vi "Event Loop Async.vi"(10 "Handshake":refnum<notifier>, 11 "ControlArray in":refnum<class "ControlArray.lvclass">) -> ()   [LabVIEW 2020, in "Control Array.lvlib" / "ControlArray.lvclass"]
uses:
  ControlArray.lvclass
  ControlArray.lvclass/ControlArray.ctl
  Element Changed Event Data.ctl
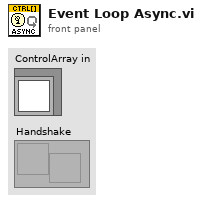
[diagram p1: front panel]
types:
  T1 = typedef "Control Array.lvlib/ControlArray.lvclass/Events.ctl" = cluster{"Stop":refnum<user-event>, "Remove Element":refnum<user-event>, "Add Element":refnum<user-event>}
  T2 = typedef "Control Array.lvlib/ControlArray.lvclass/Element Changed Event Data.ctl" = cluster{"Value":variant, "Index":i32, "Ctl Ref":refnum<vi>}
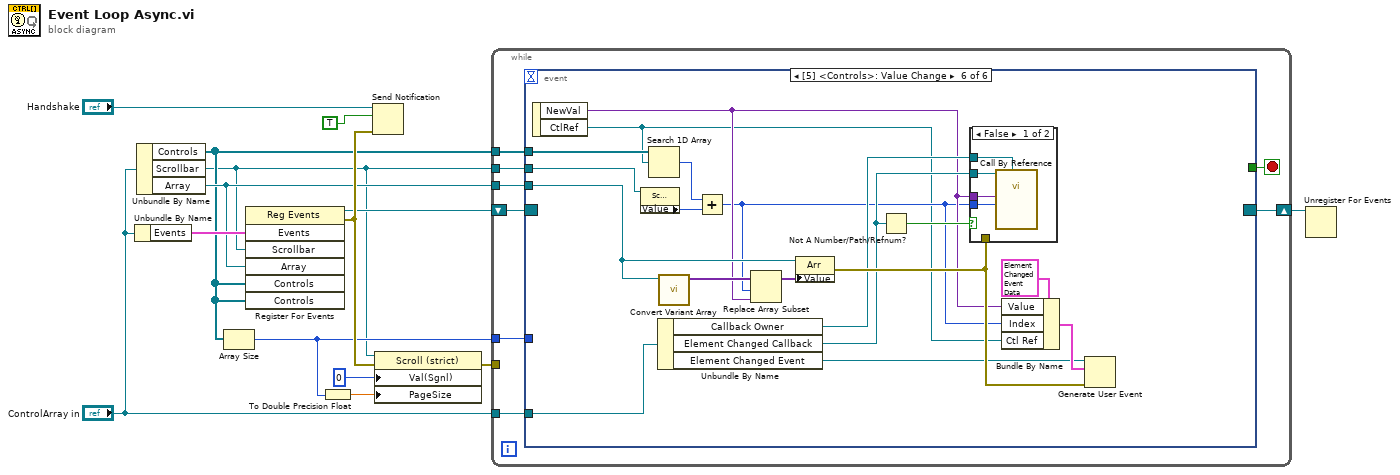
[diagram p0: block diagram]
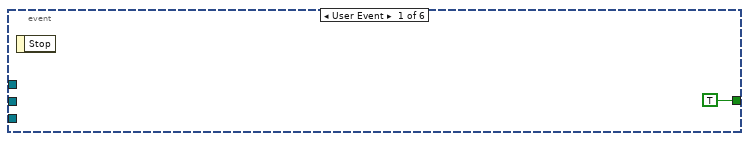
[diagram p2: hidden frame]
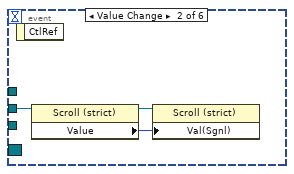
[diagram p3: hidden frame]
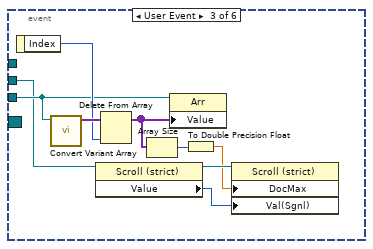
[diagram p4: hidden frame]
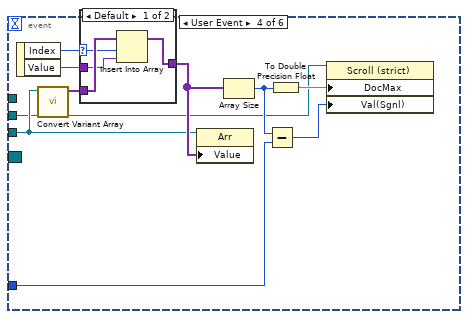
[diagram p5: hidden frame]
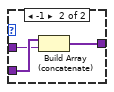
[diagram p6: hidden frame]
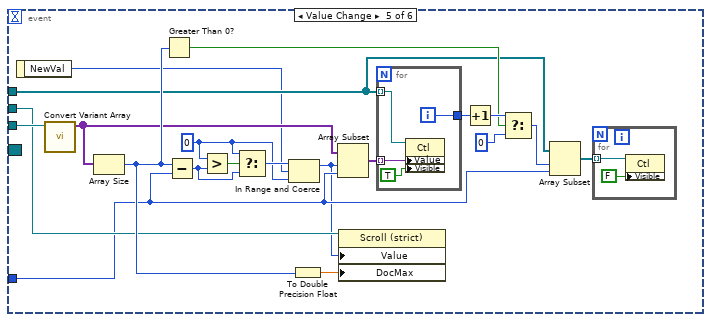
[diagram p7: hidden frame]
diagram:
  n1 = Unbundle By Name("ControlArray in") -> ("Events"=w13:T1)
  n2 = Unbundle By Name("ControlArray in") -> ("Controls"=w2:refnum<vi>[], "Scrollbar"=w1:refnum<vi>, "Array"=w7:refnum<vi>)
  n3 = Array Size(array=w2) -> (size(s)=w4:i32)
  n4 = register-events(w13, w1, w7, w2, w2) -> (reference out=w12:refnum<event-registration>, error out=w14:errorcluster)  [unwired: 2 in]
  n5 = To Double Precision Float(number=w4) -> (double precision float=w6:dbl)
  n6 = Send Notification(notification=TRUE, notifier="Handshake", error in (no error)=w14) -> ()  [unwired: 2 out]
  n7 = property class="Scroll (strict)"(reference=w1, error in=w14, "Val(Sgnl)"=0 ("Value (Signaling)"), "PageSize"=w6) -> (error out=w3:errorcluster)  [unwired: 1 out]
  n8 = while {
    shift-right: [w21] -> w11
    shift-left: w12 -> [w22]
    tunnel: w2 -> [w19]
    tunnel: w1 -> [w18]
    tunnel: w7 -> [w17]
    tunnel: "ControlArray in" -> [w16]
    tunnel: w4 -> [w15]
    tunnel: w3 -> [_]
    stop <- w20 stop-if-true
    n9 = event shown="[5] <Controls>: Value Change" {
      selector: w22 -> [_ _ _ _ _ _]
      dyn-events: [_ _ _ _ _ _] -> w21
      timeout: _ -> [_ _ _ _ _ _]
      tunnel: [TRUE _ _ _ _ _] -> w20
      tunnel: w19 -> [_ _ _ _ w55 w88]
      tunnel: w18 -> [_ w26 w27 w37 w57 w87]
      tunnel: w17 -> [_ _ w28 w38 w58 w86]
      tunnel: w16 -> [_ _ _ _ _ w85]
      tunnel: w15 -> [_ _ _ w36 w56 _]
      event User Event {
        n10 = event-data() -> ()  [unwired: 1 in, 1 out]
      }
      event Value Change {
        n11 = event-data() -> ()  [unwired: 1 in, 1 out]
        n12 = property class="Scroll (strict)"(reference=w26) -> (reference out=w25:refnum<vi>, "Value"=w24:i32)  [unwired: 1 in, 1 out]
        n13 = property class="Scroll (strict)"(reference=w25, "Val(Sgnl)"=w24) -> ()  [unwired: 1 in, 2 out]
      }
      event User Event {
        n14 = event-data() -> ("Index"=w29:i32)  [unwired: 1 in]
        n15 = call "Convert Variant Array.vi"("Array"=w28) -> ("Variant Array"=w30:variant[])  [unwired: 9 in, 1 out]
        n16 = property class="Scroll (strict)"(reference=w27) -> (reference out=w35:refnum<vi>, "Value"=w34:i32)  [unwired: 1 in, 1 out]
        n17 = Delete From Array(array=w30, index=w29) -> (array with subset deleted=w31:variant[])  [unwired: 1 in, 1 out]
        n18 = Array Size(array=w31) -> (size(s)=w32:i32)
        n19 = property class="Arr"(reference=w28, "Value"=w31) -> ()  [unwired: 1 in, 2 out]
        n20 = To Double Precision Float(number=w32) -> (double precision float=w33:dbl)
        n21 = property class="Scroll (strict)"(reference=w35, "DocMax"=w33, "Val(Sgnl)"=w34) -> ()  [unwired: 1 in, 2 out]
      }
      event User Event {
        n22 = event-data() -> ("Index"=w40:i32, "Value"=w39:variant)  [unwired: 1 in]
        n23 = call "Convert Variant Array.vi"("Array"=w38) -> ("Variant Array"=w41:variant[])  [unwired: 9 in, 1 out]
        n24 = case shown="Default" w40 {
          selector: w40 -> [w47 _]
          tunnel: w39 -> [w48 w51]
          tunnel: w41 -> [w49 w52]
          tunnel: [w46 w50] -> w45
          frame Default {
            n25 = Insert Into Array(array=w49, index=w47, new element=w48) -> (w46:variant[])
          }
          frame -1 {
            n26 = Build Array (concatenate)(w52, w51) -> (w50:variant[])
          }
        }
        n27 = property class="Arr"(reference=w38, "Value"=w45) -> ()  [unwired: 1 in, 2 out]
        n28 = Array Size(array=w45) -> (size(s)=w43:i32)
        n29 = Subtract(x=w43, y=w36) -> (x-y=w44:i32)
        n30 = To Double Precision Float(number=w43) -> (double precision float=w42:dbl)
        n31 = property class="Scroll (strict)"(reference=w37, "DocMax"=w42, "Val(Sgnl)"=w44) -> ()  [unwired: 1 in, 2 out]
      }
      event Value Change {
        w69 = 0 ("x")
        n32 = event-data() -> ("NewVal"=w54:i32)  [unwired: 1 in]
        n33 = call "Convert Variant Array.vi"("Array"=w58) -> ("Variant Array"=w59:variant[])  [unwired: 9 in, 1 out]
        n34 = Array Size(array=w59) -> (size(s)=w60:i32)
        n35 = Greater Than 0?(x=w60) -> (x > 0?=w65:bool)
        n36 = Subtract(x=w60, y=w56) -> (x-y=w71:i32)
        n37 = Greater?(x=w69, y=w71) -> (0:w72:bool)
        n38 = Select(t=w69, s=w72, f=w71) -> (s? t:f=w70:i32)
        n39 = In Range and Coerce(upper limit=w70, x=w54, lower limit=w69) -> (coerced(x)=w53:i32)  [unwired: 1 out]
        n40 = To Double Precision Float(number=w60) -> (double precision float=w61:dbl)
        n41 = Array Subset(array=w59, index=w53, length=w56) -> (w68:variant[])
        n42 = property class="Scroll (strict)"(reference=w57, "Value"=w53, "DocMax"=w61) -> ()  [unwired: 1 in, 2 out]
        n43 = for {
          tunnel: w68 -> [w77] mode=indexing
          tunnel: w55 -> [w78] mode=indexing
          tunnel: [w75] -> w67
          i -> [w75]
          n44 = property class="Ctl"(reference=w78, "Value"=w77, "Visible"=TRUE) -> ()  [unwired: 1 in, 2 out]
        }
        n45 = Increment(x=w67) -> (x+1=w66:i32)
        n46 = Select(t=w66, s=w65, f=0) -> (s? t:f=w63:i32)
        n47 = Array Subset(array=w55, index=w63, length=w56) -> (w62:refnum<vi>[])
        n48 = for {
          tunnel: w62 -> [w74] mode=indexing
          n49 = property class="Ctl"(reference=w74, "Visible"=FALSE) -> ()  [unwired: 1 in, 2 out]
        }
      }
      event Value Change {
        n50 = event-data() -> ("NewVal"=w81:variant, "CtlRef"=w79:refnum<vi>)  [unwired: 1 in]
        n51 = property class="Scroll (strict)"(reference=w87) -> ("Value"=w91:i32)  [unwired: 1 in, 2 out]
        n52 = Search 1D Array(1D array=w88, element=w79) -> (index of element=w92:i32)  [unwired: 1 in]
        n53 = Unbundle By Name(w85) -> ("Callback Owner"=w82:refnum<class>, "Element Changed Callback"=w83:refnum<vi>, "Element Changed Event"=w84:refnum<user-event>)
        n54 = call "Convert Variant Array.vi"("Array"=w86) -> ("Variant Array"=w89:variant[])  [unwired: 9 in, 1 out]
        n55 = Add(x=w92, y=w91) -> (x+y=w80:i32)
        n56 = Replace Array Subset(array=w89, new element=w81, index=w80) -> (w90:variant[])
        n57 = property class="Arr"(reference=w86, "Value"=w90) -> (error out=w96:errorcluster)  [unwired: 1 in, 1 out]
        n58 = Not A Number/Path/Refnum?(number/path/refnum=w83) -> (NaN/Path/Refnum?=w95:bool)
        n59 = case shown="False" w95 {
          tunnel: w83 -> [w98 _]
          tunnel: w81 -> [w100 _]
          tunnel: w80 -> [w99 _]
          tunnel: w82 -> [w97 _]
          tunnel: w96 -> [_ _]
          frame False {
            n60 = call-by-ref "?"(reference=w98, "Owner"=w97, "Index"=w99, "Value"=w100) -> ()  [unwired: 10 in, 2 out]
          }
          frame True {
          }
        }
        n61 = Bundle By Name(cluster=T2 {"Value"=variant, "Index"=0, "Ctl Ref"=refnum} ("event data"), "Value"=w81, "Index"=w80, "Ctl Ref"=w79) -> (w93:T2)
        n62 = Generate User Event(user event=w84, event data cluster=w93, error in=w96) -> ()  [unwired: 1 in, 2 out]
      }
    }
  }
  n63 = Unregister For Events(event registration refnum=w11) -> ()  [unwired: 1 in, 1 out]
